vi "background process.vi"(11 "Runtime":refnum<class "asynchronous execution module runtime.lvclass">) -> (0 "error out":errorcluster)   [LabVIEW 2013, in "asynchronous execution module runtime.lvclass"]
uses:
  asynchronous execution module runtime.lvclass
  asynchronous execution module runtime.lvclass/asynchronous execution module runtime.ctl
  <vilib>/NI/Tag Bus Module Framework/runtime/TBM module execution interface.lvclass
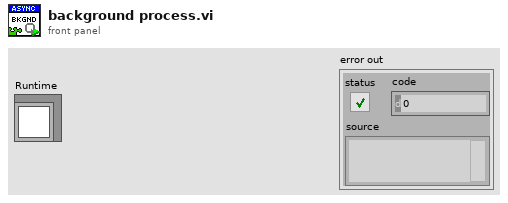
[diagram p1: front panel]
types:
  T1 = typedef "tag bus.lvlib/data table.lvlib/data table.ctl" = cluster{"Double":dbl[], "Single":sgl[], "I64":i64[], "I32":i32[], "I16":i16[], "I8":i8[], "U64":u64[], "U32":u32[], "U16":u16[], "U8":u8[], "Boolean":bool[], "String":string[], "Array of Double":cluster{"DBL Array":dbl[]}[], "Array of Single":cluster{"SGL Array":sgl[]}[], "Array of I64":cluster{"I64 Array":i64[]}[], "Array of I32":cluster{"I32 Array":i32[]}[], "Array of I16":cluster{"I16 Array":i16[]}[], "Array of I8":cluster{"I8 Array":i8[]}[], "Array of U64":cluster{"U64 Array":u64[]}[], "Array of U32":cluster{"U32 Array":u32[]}[], "Array of U16":cluster{"U16 Array":u16[]}[], "Array of U8":cluster{"U8 Array":u8[]}[], "Array of Boolean":cluster{"Boolean Array":bool[]}[], "Array of String":cluster{"String Array":string[]}[]}
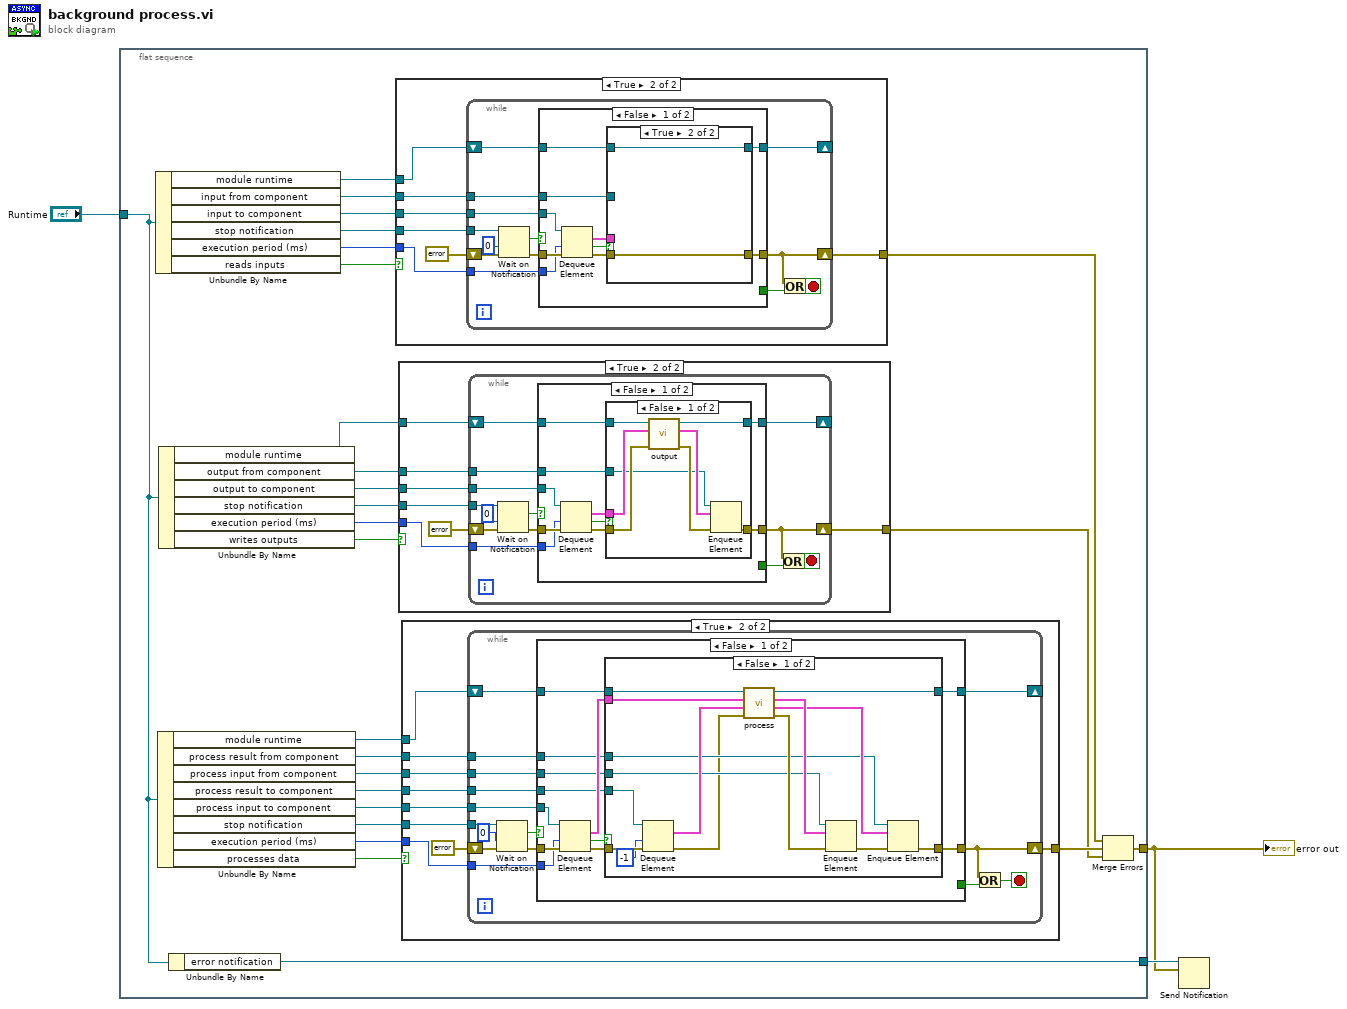
[diagram p0: block diagram]
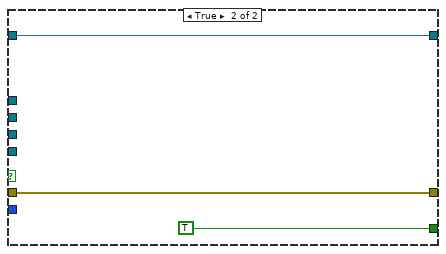
[diagram p4: hidden frame]
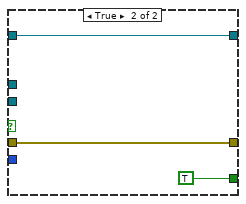
[diagram p7: hidden frame]
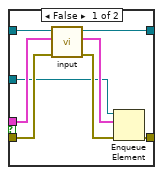
[diagram p9: hidden frame]
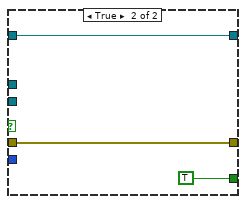
[diagram p10: hidden frame]
diagram:
  n1 = flat-sequence {
    tunnel: "Runtime" -> [w9]
    tunnel: [w15] -> w2
    tunnel: [w11] -> w1
    frame #0 {
      n2 = Unbundle By Name(w9) -> ("module runtime"=w8:refnum<class "TBM module execution interface.lvclass">, "input from component"=w26:refnum<queue>, "input to component"=w27:refnum<queue>, "stop notification"=w29:refnum<notifier>, "execution period (ms)"=w28:i32, "reads inputs"=w6:bool)
      n3 = Unbundle By Name(w9) -> ("module runtime"=w7:refnum<class "TBM module execution interface.lvclass">, "process result from component"=w17:refnum<queue>, "process input from component"=w16:refnum<queue>, "process result to component"=w18:refnum<queue>, "process input to component"=w19:refnum<queue>, "stop notification"=w21:refnum<notifier>, "execution period (ms)"=w20:i32, "processes data"=w4:bool)
      n4 = Unbundle By Name(w9) -> ("module runtime"=w10:refnum<class "TBM module execution interface.lvclass">, "output from component"=w25:refnum<queue>, "output to component"=w24:refnum<queue>, "stop notification"=w22:refnum<notifier>, "execution period (ms)"=w23:i32, "writes outputs"=w5:bool)
      n5 = Unbundle By Name(w9) -> ("error notification"=w15:refnum<notifier>)
      n6 = case shown="True" w6 {
        tunnel: w29 -> [_ w135]
        tunnel: w28 -> [_ w134]
        tunnel: w27 -> [_ w133]
        tunnel: w26 -> [_ w132]
        tunnel: [_ w130] -> w13
        tunnel: w8 -> [_ w129]
        frame False {
        }
        frame True {
          n7 = while {
            tunnel: w135 -> [w148]
            tunnel: w134 -> [w140]
            shift-right: [w145] -> _
            shift-left: w129 -> [w146]
            shift-right: [w143] -> w130
            shift-left: errorcluster {"status"=FALSE, "code"=0, "source"=""} ("error out") -> [w144]
            tunnel: w133 -> [w139]
            tunnel: w132 -> [w138]
            stop <- w141 stop-if-true
            n8 = Wait on Notification(notifier=w148, timeout in ms (-1)=0, error in (no error)=w144) -> (notification=w136:bool, error out=w147:errorcluster)  [unwired: 1 in, 2 out]
            n9 = case shown="False" w136 {
              tunnel: w147 -> [w156 w171]
              tunnel: w146 -> [w158 w169]
              tunnel: [w157 w169] -> w145
              tunnel: [w152 w171] -> w143
              tunnel: [_ TRUE] -> w142
              tunnel: w140 -> [w149 _]
              tunnel: w139 -> [w155 _]
              tunnel: w138 -> [w151 _]
              frame False {
                n10 = Dequeue Element(queue=w155, timeout in ms (-1)=w149, error in (no error)=w156) -> (element=w154:T1, timed out?=w150:bool, error out=w153:errorcluster)  [unwired: 1 out]
                n11 = case shown="True" w150 {
                  tunnel: w158 -> [w166 w168]
                  tunnel: [w165 w168] -> w157
                  tunnel: w154 -> [w164 _]
                  tunnel: w153 -> [w163 w167]
                  tunnel: [w162 w167] -> w152
                  tunnel: w151 -> [w159 _]
                  frame False {
                    n12 = call-dynamic "input.vi"("error in"=w163, "input allocation"=w164, "module in"=w166) -> ("error out"=w161:errorcluster, "input data"=w160:T1, "module out"=w165:refnum<class "TBM module execution interface.lvclass">)  [unwired: 6 in]
                    n13 = Enqueue Element(queue=w159, element=w160, error in (no error)=w161) -> (error out=w162:errorcluster)  [unwired: 1 in, 2 out]
                  }
                  frame True {
                  }
                }
              }
              frame True {
              }
            }
            n14 = Or(x=w143, y=w142) -> (x .or. y?=w141:bool)
          }
        }
      }
      n15 = case shown="True" w5 {
        tunnel: w25 -> [_ w91]
        tunnel: w24 -> [_ w90]
        tunnel: w23 -> [_ w89]
        tunnel: w22 -> [_ w88]
        tunnel: [_ w87] -> w12
        tunnel: w10 -> [_ w86]
        frame False {
        }
        frame True {
          n16 = while {
            tunnel: w88 -> [w105]
            tunnel: w89 -> [w97]
            shift-right: [w102] -> _
            shift-left: w86 -> [w103]
            shift-right: [w100] -> w87
            shift-left: errorcluster {"status"=FALSE, "code"=0, "source"=""} ("error out") -> [w101]
            tunnel: w90 -> [w96]
            tunnel: w91 -> [w95]
            stop <- w98 stop-if-true
            n17 = Wait on Notification(notifier=w105, timeout in ms (-1)=0, error in (no error)=w101) -> (notification=w93:bool, error out=w104:errorcluster)  [unwired: 1 in, 2 out]
            n18 = case shown="False" w93 {
              tunnel: w104 -> [w113 w128]
              tunnel: w103 -> [w115 w126]
              tunnel: [w114 w126] -> w102
              tunnel: [w109 w128] -> w100
              tunnel: [_ TRUE] -> w99
              tunnel: w97 -> [w106 _]
              tunnel: w96 -> [w112 _]
              tunnel: w95 -> [w108 _]
              frame False {
                n19 = Dequeue Element(queue=w112, timeout in ms (-1)=w106, error in (no error)=w113) -> (element=w111:T1, timed out?=w107:bool, error out=w110:errorcluster)  [unwired: 1 out]
                n20 = case shown="False" w107 {
                  tunnel: w115 -> [w123 w125]
                  tunnel: [w122 w125] -> w114
                  tunnel: w111 -> [w121 _]
                  tunnel: w110 -> [w120 w124]
                  tunnel: [w119 w124] -> w109
                  tunnel: w108 -> [w116 _]
                  frame False {
                    n21 = call-dynamic "output.vi"("error in"=w120, "output data"=w121, "module in"=w123) -> ("error out"=w118:errorcluster, "output allocation"=w117:T1, "module out"=w122:refnum<class "TBM module execution interface.lvclass">)  [unwired: 6 in]
                    n22 = Enqueue Element(queue=w116, element=w117, error in (no error)=w118) -> (error out=w119:errorcluster)  [unwired: 1 in, 2 out]
                  }
                  frame True {
                  }
                }
              }
              frame True {
              }
            }
            n23 = Or(x=w100, y=w99) -> (x .or. y?=w98:bool)
          }
        }
      }
      n24 = case shown="True" w4 {
        tunnel: w21 -> [_ w38]
        tunnel: w20 -> [_ w37]
        tunnel: w19 -> [_ w35]
        tunnel: w18 -> [_ w34]
        tunnel: w17 -> [_ w33]
        tunnel: w16 -> [_ w32]
        tunnel: [_ w31] -> w14
        tunnel: w7 -> [_ w30]
        frame False {
        }
        frame True {
          n25 = while {
            tunnel: w38 -> [w53]
            tunnel: w37 -> [w45]
            shift-right: [w50] -> _
            shift-left: w30 -> [w51]
            shift-right: [w48] -> w31
            shift-left: errorcluster {"status"=FALSE, "code"=0, "source"=""} ("error out") -> [w49]
            tunnel: w35 -> [w44]
            tunnel: w34 -> [w43]
            tunnel: w33 -> [w42]
            tunnel: w32 -> [w41]
            stop <- w46 stop-if-true
            n26 = Wait on Notification(notifier=w53, timeout in ms (-1)=0, error in (no error)=w49) -> (notification=w39:bool, error out=w52:errorcluster)  [unwired: 1 in, 2 out]
            n27 = case shown="False" w39 {
              tunnel: w52 -> [w63 w85]
              tunnel: w51 -> [w65 w83]
              tunnel: [w64 w83] -> w50
              tunnel: [w60 w85] -> w48
              tunnel: [_ TRUE] -> w47
              tunnel: w45 -> [w56 _]
              tunnel: w44 -> [w58 _]
              tunnel: w43 -> [w57 _]
              tunnel: w42 -> [w55 _]
              tunnel: w41 -> [w54 _]
              frame False {
                n28 = Dequeue Element(queue=w58, timeout in ms (-1)=w56, error in (no error)=w63) -> (element=w62:T1, timed out?=w59:bool, error out=w61:errorcluster)  [unwired: 1 out]
                n29 = case shown="False" w59 {
                  tunnel: w65 -> [w80 w82]
                  tunnel: [w79 w82] -> w64
                  tunnel: w62 -> [w72 _]
                  tunnel: w61 -> [w75 w81]
                  tunnel: [w77 w81] -> w60
                  tunnel: w57 -> [w74 _]
                  tunnel: w55 -> [w68 _]
                  tunnel: w54 -> [w67 _]
                  frame False {
                    n30 = Dequeue Element(queue=w74, timeout in ms (-1)=-1, error in (no error)=w75) -> (element=w71:T1, error out=w66:errorcluster)  [unwired: 2 out]
                    n31 = call-dynamic "process.vi"("error in"=w66, "result allocation"=w71, "parameters"=w72, "module in"=w80) -> ("error out"=w78:errorcluster, "results"=w69:T1, "parameter allocation"=w70:T1, "module out"=w79:refnum<class "TBM module execution interface.lvclass">)  [unwired: 4 in]
                    n32 = Enqueue Element(queue=w67, element=w70, error in (no error)=w78) -> (error out=w76:errorcluster)  [unwired: 1 in, 2 out]
                    n33 = Enqueue Element(queue=w68, element=w69, error in (no error)=w76) -> (error out=w77:errorcluster)  [unwired: 1 in, 2 out]
                  }
                  frame True {
                  }
                }
              }
              frame True {
              }
            }
            n34 = Or(x=w48, y=w47) -> (x .or. y?=w46:bool)
          }
        }
      }
      n35 = Merge Errors(w13, w14, w12) -> (w11:errorcluster)
    }
  }
  n36 = Send Notification(notification=w1, notifier=w2) -> ()  [unwired: 1 in, 2 out]
  "error out" <- w1
